vi "conv-src_vers_src-aff.vi"() -> (4 "src_aff":T18, 6 "stat-aff":T17 caption="Stat. V")   [LabVIEW 2010, in "lv_04.lvlib"]
uses:
  lv_04/lv_04.lvlib
  lv_04/commandes/cSTA-C-aff.ctl
  lv_04/commandes/c_TDMS_ch_donnees.ctl
  lv_04/commandes/c_TDMS_ch_variable.ctl
  lv_04/commandes/c0-var-n.ctl
  lv_04/commandes/cSTA-C-cs.ctl
  lv_04/commandes/cX.ctl
  lv_04/commandes/cSTA_varid.ctl
  lv_04/commandes/cSTA_num_do_cr.ctl
  lv_04/commandes/c02-do-num.ctl
  lv_04/commandes/c04-stat-num.ctl
  lv_04/commandes/cSTA_txt_do_cr.ctl
  lv_04/commandes/c02-do-txt.ctl
  lv_04/commandes/c04-stat-txt.ctl
  lv_04/commandes/cSTA_dist.ctl
  lv_04/commandes/c03-dist-S.ctl
  lv_04/commandes/c0-dist-xy.ctl
  lv_04/commandes/c03-dist-T.ctl
  lv_04/commandes/c03-dist-SPC.ctl
panel:
  in  "cX":T1
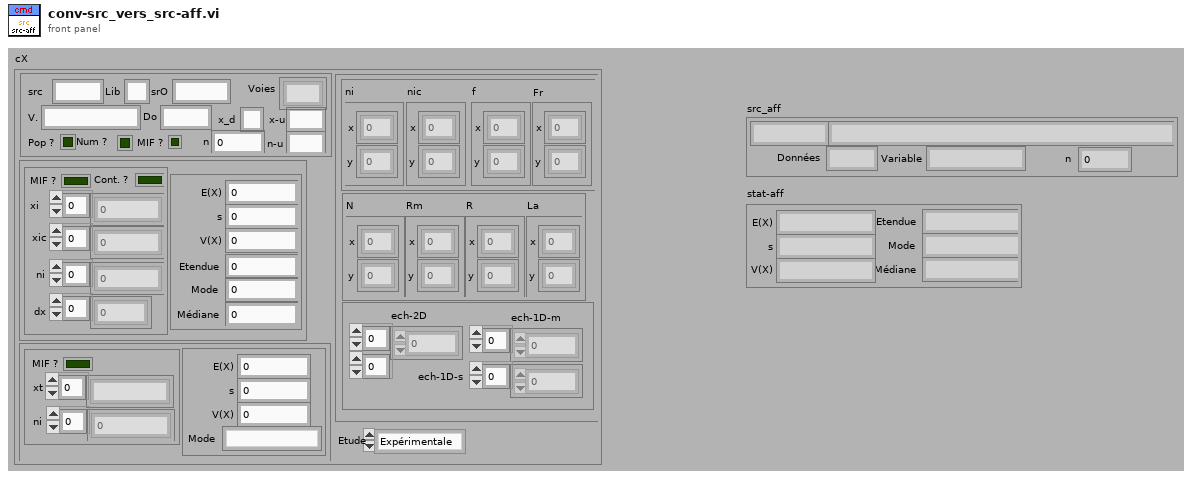
[diagram p1: front panel]
types:
  T1 = typedef "lv_04.lvlib/cX.ctl" = cluster{"src":T2, "num":T6, "txt":T9, "dist":T12, "Etude":enum16{"Expérimentale", "Modèle"}}
  T2 = typedef "lv_04.lvlib/cSTA_varid.ctl" = cluster{"src":string, "Lib":string, "srO":string, "V.":T3, "Voies":string[], "Do":T4, "n":T5, "Num ?":bool, "Pop ?":bool, "x_d":string, "x-u":string, "n-u":string, "MIF ?":bool}
  T3 = typedef "lv_04.lvlib/c_TDMS_ch_variable.ctl" = string
  T4 = typedef "lv_04.lvlib/c_TDMS_ch_donnees.ctl" = string
  T5 = typedef "lv_04.lvlib/c0-var-n.ctl" = i32
  T6 = typedef "lv_04.lvlib/cSTA_num_do_cr.ctl" = cluster{"do":T7, "sta":T8}
  T7 = typedef "lv_04.lvlib/c02-do-num.ctl" = cluster{"MIF ?":bool, "Cont. ?":bool, "xi":dbl[], "xic":dbl[], "ni":u32[], "dx":dbl[]}
  T8 = typedef "lv_04.lvlib/c04-stat-num.ctl" = cluster{"E(X)":dbl, "s":dbl, "V(X) ":dbl, "Etendue":dbl, "Mode":dbl, "Médiane":dbl}
  T9 = typedef "lv_04.lvlib/cSTA_txt_do_cr.ctl" = cluster{"do":T10, "sta":T11}
  T10 = typedef "lv_04.lvlib/c02-do-txt.ctl" = cluster{"xt":string[], "ni":dbl[], "MIF ?":bool}
  T11 = typedef "lv_04.lvlib/c04-stat-txt.ctl" = cluster{"E(X)":dbl, "s":dbl, "V(X) ":dbl, "Mode":string}
  T12 = typedef "lv_04.lvlib/cSTA_dist.ctl" = cluster{"S":T13, "T":T15, "spc":T16}
  T13 = typedef "lv_04.lvlib/c03-dist-S.ctl" = cluster{"nic":T14, "f":T14, "Fr":T14, "ni":T14}
  T14 = typedef "lv_04.lvlib/c0-dist-xy.ctl" = cluster{"x":dbl[], "y":dbl[]}
  T15 = typedef "lv_04.lvlib/c03-dist-T.ctl" = cluster{"N":T14, "Rm":T14, "R":T14, "La":T14}
  T16 = typedef "lv_04.lvlib/c03-dist-SPC.ctl" = cluster{"ech-2D":dbl[][], "ech-1D-m":dbl[], "ech-1D-s":dbl[]}
  T17 = typedef "lv_04.lvlib/cSTA-C-cs.ctl" = cluster{"E(X)":string, "s":string, "V(X) ":string, "Mode":string, "Médiane":string, "Etendue":string}
  T18 = typedef "lv_04.lvlib/cSTA-C-aff.ctl" = cluster{"src":string, "Lib":string, "Données":T4, "Variable":T3, "n":T5}
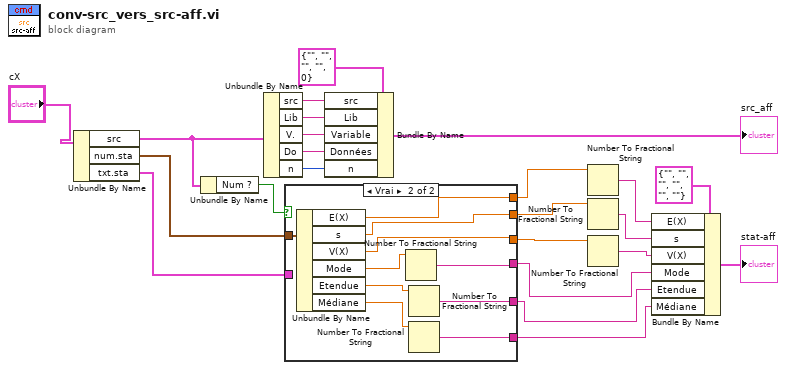
[diagram p0: block diagram]
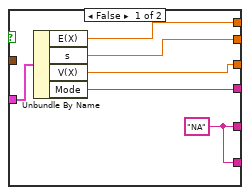
[diagram p2: hidden frame]
diagram:
  n1 = Unbundle By Name("cX") -> ("src"=w16:T2, "num.sta"=w12:T8, "txt.sta"=w5:T11)
  n2 = Unbundle By Name(w16) -> ("Num ?"=w15:bool)
  n3 = Unbundle By Name(w16) -> ("src"=w18:string, "Lib"=w19:string, "V."=w20:T3, "Do"=w21:T4, "n"=w22:T5)
  n4 = case shown="Vrai" w15 {
    tunnel: w12 -> [_ w39]
    tunnel: [w29 w38] -> w11
    tunnel: [w28 w37] -> w9
    tunnel: [w27 w36] -> w7
    tunnel: w5 -> [w26 _]
    tunnel: [w25 w34] -> w4
    tunnel: [w24 w32] -> w3
    tunnel: [w24 w30] -> w2
    frame False {
      w24 = "NA"
      n5 = Unbundle By Name(w26) -> ("E(X)"=w29:dbl, "s"=w28:dbl, "V(X)"=w27:dbl, "Mode"=w25:string)
    }
    frame True {
      n6 = Unbundle By Name(w39) -> ("E(X)"=w38:dbl, "s"=w37:dbl, "V(X)"=w36:dbl, "Mode"=w35:dbl, "Etendue"=w33:dbl, "Médiane"=w31:dbl)
      n7 = Number To Fractional String(number=w35) -> (F-format string=w34:string)  [unwired: 3 in]
      n8 = Number To Fractional String(number=w33) -> (F-format string=w32:string)  [unwired: 3 in]
      n9 = Number To Fractional String(number=w31) -> (F-format string=w30:string)  [unwired: 3 in]
    }
  }
  n10 = Bundle By Name(cluster=T18 {"src"="", "Lib"="", "Données"="", "Variable"="", "n"=0} ("src_aff"), "src"=w18, "Lib"=w19, "Variable"=w20, "Données"=w21, "n"=w22) -> (→"src_aff":T18)
  n11 = Number To Fractional String(number=w11) -> (F-format string=w10:string)  [unwired: 3 in]
  n12 = Number To Fractional String(number=w9) -> (F-format string=w8:string)  [unwired: 3 in]
  n13 = Number To Fractional String(number=w7) -> (F-format string=w6:string)  [unwired: 3 in]
  n14 = Bundle By Name(cluster=T17 {"E(X)"="", "s"="", "V(X) "="", "Mode"="", "Médiane"="", "Etendue"=""} ("stat-aff 2"), "E(X)"=w10, "s"=w8, "V(X)"=w6, "Mode"=w4, "Etendue"=w3, "Médiane"=w2) -> (→"stat-aff":T17)
